vi "断电保存全局.vi"() -> ()   [LabVIEW 2016]
panel:
  in  "connection information":string="mysql"
  out "配置表格":string[][](table)
  out "因子编码簇":T1
  in  "QYMC":string="安徽晨蓝环保科技有限公司（凤台经济开发区污水处理厂）"
  in  "QYBH":string="340100000133"
  in  "PKMC":string="污水排口"
  in  "PKBH":string="340400000010WaterOutput2"
  in  "XH":string="34040000001020012018103012"
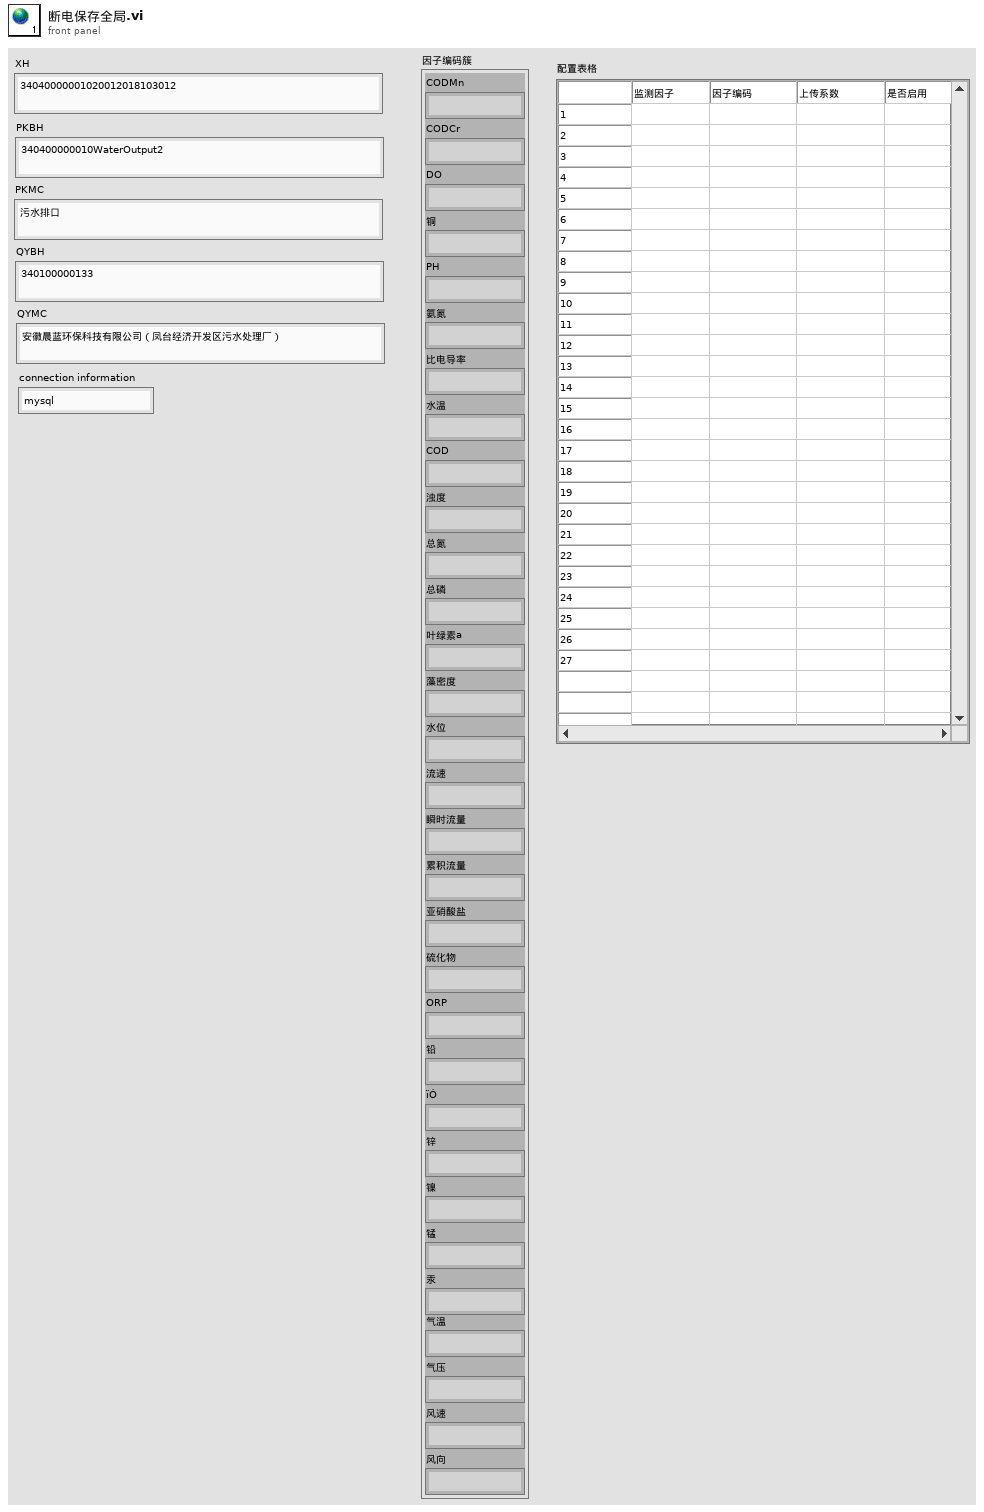
[diagram p1: front panel]
types:
  T1 = cluster{"CODMn":string, "CODCr":string, "DO":string, "铜":string, "PH":string, "氨氮":string, "比电导率":string, "水温":string, "COD":string, "浊度":string, "总氮":string, "总磷":string, "叶绿素a":string, "藻密度":string, "水位":string, "流速":string, "瞬时流量":string, "累积流量":string, "亚硝酸盐":string, "硫化物":string, "ORP":string, "铅":string, "ïÓ":string, "锌":string, "镍":string, "锰":string, "汞":string, "气温":string, "气压":string, "风速":string, "风向":string}
diagram:
